vi "test_Checksum U16 - Check Protection with corrupt data.vi"(8 "error in (no error)":errorcluster) -> (0 "error out":errorcluster)   [LabVIEW 2019, in "Protections Unit Tests.lvclass"]
uses:
  Protections Unit Tests.lvclass
  Checksum U16/Checksum U16.lvclass
  64e6d109-6c77-4232-8703-168182d74ffb.vi
  <vilib>/addons/_JKI Toolkits/VI Tester/TestCase.llb/TestCase.lvclass
  C:/Program Files (x86)/National Instruments/LabVIEW 2019/vi.lib/addons/_JKI Toolkits/VI Tester/TestCase.llb/TestCase.lvclass
panel:
  out "Checksum U16 out":refnum<class "Checksum U16.lvclass">
  in  "Checksum U16 in":refnum<class "Checksum U16.lvclass">
  out "TestCase out":refnum<class "Protections Unit Tests.lvclass">
  in  "TestCase in":refnum<class "Protections Unit Tests.lvclass">
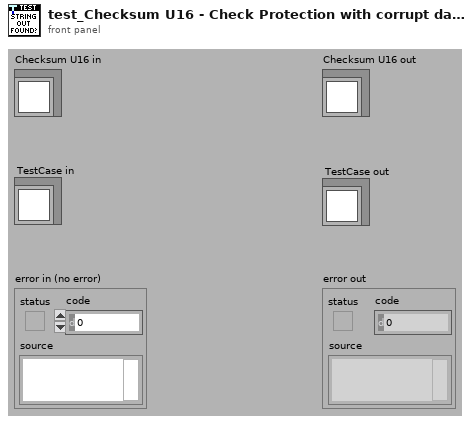
[diagram p1: front panel]
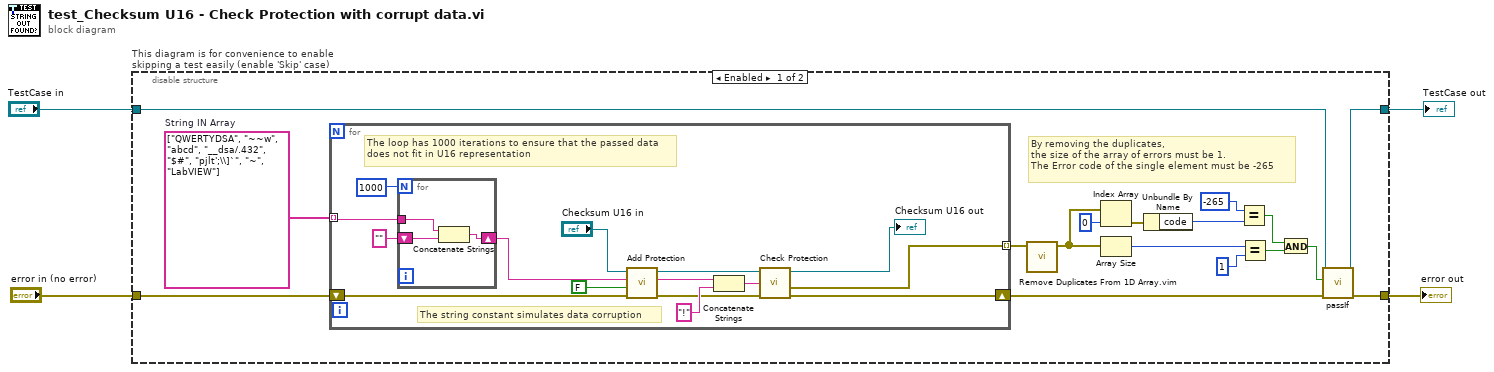
[diagram p0: block diagram]
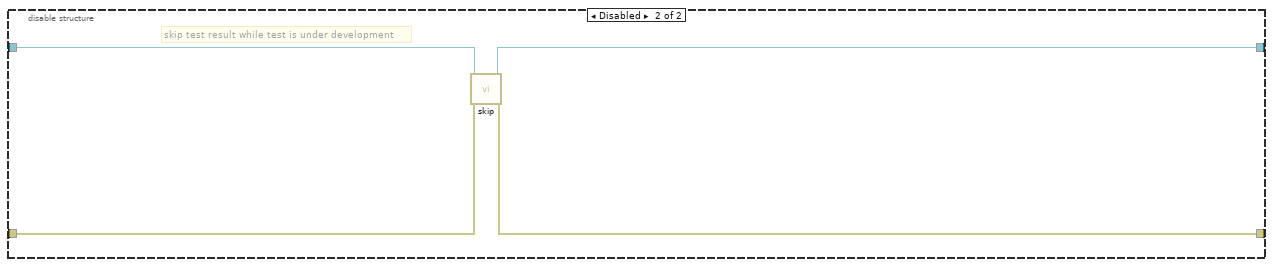
[diagram p2: hidden frame]
diagram:
  n1 = disable-structure "This diagram is for convenience to enable skipping a test easily (enable 'Skip' case)" shown="Enabled" {
    disable-tunnel: "TestCase in" -> [w19 w43]
    disable-tunnel: [w18 w41] -> w1
    disable-tunnel: [w17 w42] -> w3
    disable-tunnel: "error in (no error)" -> [w21 w40]
    frame Enabled {
      w20 = string[] ["QWERTYDSA", "~~w", "abcd", "__dsa/.432", "$#", "pjlt';\\]`", "~", "LabVIEW"]  # String IN Array
      # "By removing the duplicates, \nthe size of the array of errors must be 1. \nThe Error code of the single element must be -265"
      n2 = for {
        tunnel: w20 -> [w34] mode=indexing
        shift-right: [w22] -> w16
        shift-left: w21 -> [w32]
        tunnel: [w23] -> w5 mode=indexing
        # "The string constant simulates data corruption"
        # "The loop has 1000 iterations to ensure that the passed data\ndoes not fit in U16 representation"
        n3 = for {
          N: 1000 -> [_]
          shift-right: [w39] -> w30
          shift-left: "" -> [w38]
          tunnel: w34 -> [w37]
          n4 = Concatenate Strings(w37, w38) -> (w39:string)
        }
        n5 = call-dynamic "Add Protection.vi"("error in (no error)"=w32, "Pad"=FALSE, "String in"=w30, "Checksum U16 in"="Checksum U16 in") -> ("error out"=w26:errorcluster, "String out"=w28:string, "Checksum U16 out"=w27:refnum<class "Checksum U16.lvclass">)  [unwired: 5 in]
        n6 = Concatenate Strings(w28, "!" ("string")) -> (w25:string)
        n7 = call-dynamic "Check Protection.vi"("error in (no error)"=w26, "String in"=w25, "Checksum U16 in"=w27) -> ("error out"=w22:errorcluster, "Protection Error"=w23:errorcluster, "Checksum U16 out"=→"Checksum U16 out":refnum<class "Checksum U16.lvclass">)  [unwired: 5 in, 1 out]
      }
      n8 = call "Remove Duplicates From 1D Array.vim"("array"=w5) -> ("array with duplicates removed"=w10:errorcluster[])  [unwired: 10 in]
      n9 = Index Array(array=w10, index=0) -> (element=w8:errorcluster)
      n10 = Array Size(array=w10) -> (size(s)=w15:i32)
      n11 = Unbundle By Name(w8) -> ("code"=w7:i32)
      n12 = Equal?(x=-265, y=w7) -> (x = y?=w12:bool)
      n13 = Equal?(x=w15, y=1) -> (x = y?=w11:bool)
      n14 = And(x=w12, y=w11) -> (x .and. y?=w6:bool)
      n15 = call-dynamic "passIf.vi"("error in (no error)"=w16, "pass"=w6, "TestCase in"=w19) -> ("error out"=w17:errorcluster, "TestCase out"=w18:refnum<class "Protections Unit Tests.lvclass">)  [unwired: 7 in]
    }
    frame Disabled {
      # "skip test result while test is under development"
      n16 = call <vilib>:"skip.vi"("error in (no error)"=w40, "TestCase in"=w43) -> ("error out"=w42:errorcluster, "TestCase out"=w41:refnum<class "Protections Unit Tests.lvclass">)  [unwired: 8 in]
    }
  }
  "error out" <- w3
  "TestCase out" <- w1
